vi "TurretEncoderToAngle.vi"(11 "encoderPulses":i32) -> (3 "angle(deg)":dbl)   [LabVIEW 2018]
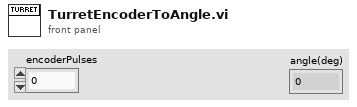
[diagram p1: front panel]
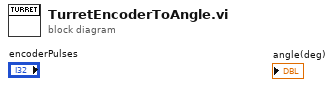
[diagram p0: block diagram]
diagram:
